vi "air pressure setting.vi"() -> (0 "air pressure indecator":i32, 1 "deposit speed 2":dbl)   [LabVIEW 2016]
panel:
  in  "deposit speed":dbl=10.0
  in  "start applying glue":bool
  in  "air pressure":i32=20
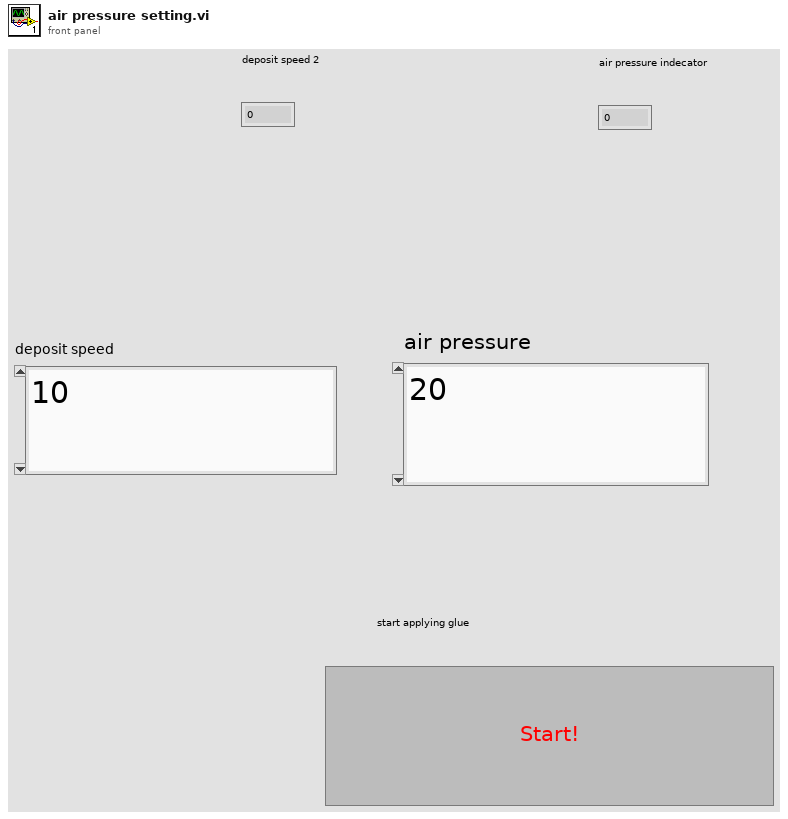
[diagram p1: front panel]
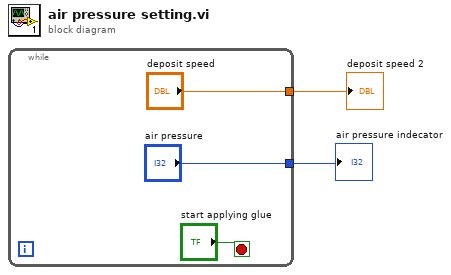
[diagram p0: block diagram]
diagram:
  n1 = while {
    tunnel: ["air pressure"] -> w2
    tunnel: ["deposit speed"] -> w1
    stop <- "start applying glue" stop-if-true
  }
  "air pressure indecator" <- w2
  "deposit speed 2" <- w1
